vi "VeriStand DSF.Plugin.Configuration.Create.vi"(8 "error in (no error)":errorcluster, 10 "Section Ref":T1=18446744073709551615 format="%.0x", 11 "Device Ref":T1=18446744073709551615 format="%.0x") -> (0 "error out":errorcluster, 3 "Plugin Configuration":refnum<class "VeriStand DSF.Plugin.Configuration.lvclass">)   [LabVIEW 2017, in "Data Sharing Custom Device Engine.lvlib" / "VeriStand DSF.Plugin.Configuration.lvclass"]
uses:
  VeriStand DSF.Plugin.Configuration.lvclass
  <vilib>/NI Veristand/Custom Device API/Custom Device Item Ref.ctl
  VeriStand DSF.Plugin.Configuration.lvclass/VeriStand DSF.Plugin.Configuration.ctl
  VeriStand DSF.Transfer Group.Configuration.lvclass
  C:/Builds/Data Sharing Framework/Current/Data Sharing Framework Core/DSF Core.lvlibp/Shared/Classes/Transfer Group/Transfer Group Configuration.lvclass
  <vilib>/NI Veristand/Custom Device API/Custom Device API.lvlib
  Builds/Data Sharing Framework/Current/Data Sharing Framework Core/DSF Core.lvlibp/Shared/Classes/Plugin/Plugin Configuration.lvclass
  C:/Builds/Data Sharing Framework/Current/Data Sharing Framework Core/DSF Core.lvlibp/Shared/Classes/Plugin/Plugin Configuration.lvclass
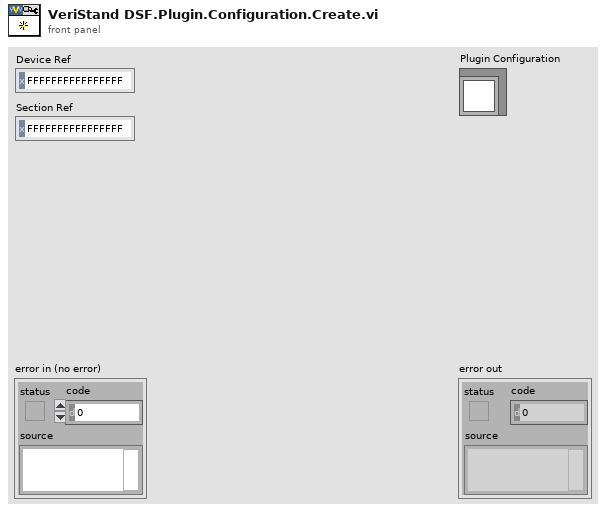
[diagram p1: front panel]
types:
  T1 = typedef "Custom Device API.lvlib/Custom Device Item Ref.ctl" = u64
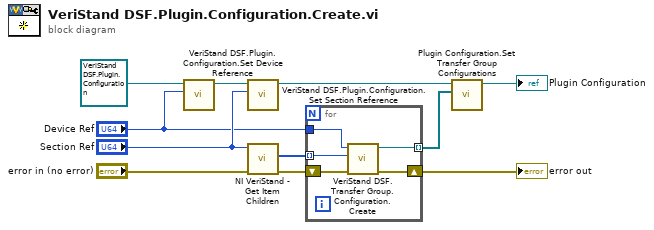
[diagram p0: block diagram]
diagram:
  n1 = call "VeriStand DSF.Plugin.Configuration.Set Device Reference.vi"("Device Ref"="Device Ref", "VeriStand DSF.Plugin.Configuration in"=refnum<class "VeriStand DSF.Plugin.Configuration.lvclass"> refnum ("VeriStand DSF.Plugin.Configuration.lvclass")) -> ("VeriStand DSF.Plugin.Configuration out"=w3:refnum<class "VeriStand DSF.Plugin.Configuration.lvclass">)  [unwired: 9 in]
  n2 = call "VeriStand DSF.Plugin.Configuration.Set Section Reference.vi"("Section Ref"="Section Ref", "VeriStand DSF.Plugin.Configuration in"=w3) -> ("VeriStand DSF.Plugin.Configuration out"=w11:refnum<class "VeriStand DSF.Plugin.Configuration.lvclass">)  [unwired: 9 in]
  n3 = call <vilib>:"NI VeriStand - Get Item Children.vi"("error in (no error)"="error in (no error)", "Item Ref in"="Section Ref") -> ("error out"=w7:errorcluster, "Child Refs"=w4:T1[])  [unwired: 6 in, 2 out]
  n4 = for {
    shift-right: [w15] -> w5
    shift-left: w7 -> [w16]
    tunnel: w4 -> [w13] mode=indexing
    tunnel: [w14] -> w6 mode=indexing
    tunnel: "Device Ref" -> [w12]
    n5 = call "VeriStand DSF.Transfer Group.Configuration.Create.vi"("error in (no error)"=w16, "Section Ref"=w13, "Device Ref"=w12) -> ("error out"=w15:errorcluster, "Transfer Group Configuration"=w14:refnum<class "VeriStand DSF.Transfer Group.Configuration.lvclass">)  [unwired: 7 in]
  }
  "error out" <- w5
  n6 = call "Plugin Configuration.Set Transfer Group Configurations.vi"("Transfer Group Configurations"=w6, "Plugin Configuration in"=w11) -> ("Plugin Configuration out"=→"Plugin Configuration":refnum<class "VeriStand DSF.Plugin.Configuration.lvclass">)  [unwired: 9 in]
